vi "Get Recipe Version.vi"(8 "error in (no error)":errorcluster, 11 "Test Recipe in":refnum<class "Test Recipe.lvclass">) -> (0 "error out":errorcluster, 2 "Test Recipe Version":string, 3 "Test Recipe out":refnum<class "Test Recipe.lvclass">)   [LabVIEW 2015, in "Test Recipe.lvlib" / "Test Recipe.lvclass"]
doc: "Searches for a recipe version and retrieves it. Returns \"9.9.9.9\" if no version exists."
uses:
  Test Recipe.lvclass
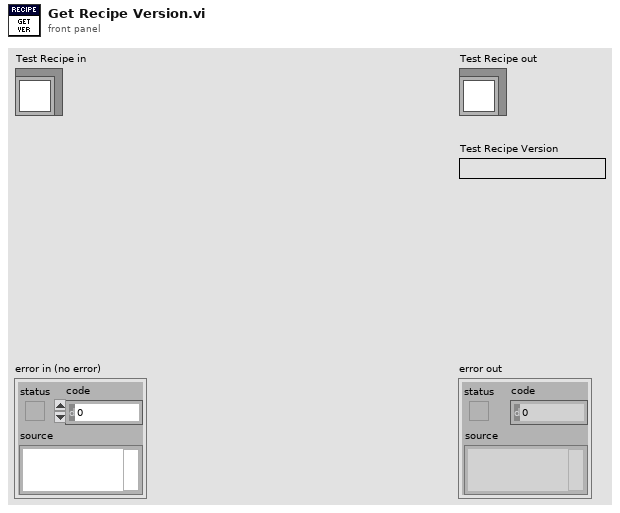
[diagram p1: front panel]
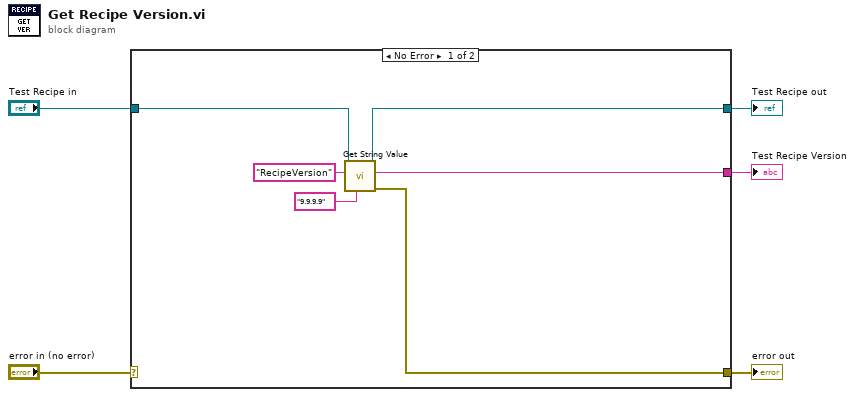
[diagram p0: block diagram]
diagram:
  n1 = case shown="No Error" "error in (no error)" {
    selector: "error in (no error)" -> [_ w13]
    tunnel: [w6 w13] -> w4
    tunnel: [w10 w12] -> w2
    tunnel: "Test Recipe in" -> [w11 w12]
    tunnel: [w7 _] -> w1
    frame No Error {
      n2 = call "Get String Value.vi"("Default Value"="9.9.9.9", "Name"="RecipeVersion", "Test Recipe in"=w11) -> ("error out"=w6:errorcluster, "Value"=w7:string, "Test Recipe out"=w10:refnum<class "Test Recipe.lvclass">)  [unwired: 6 in]
    }
    frame Error {
    }
  }
  "error out" <- w4
  "Test Recipe out" <- w2
  "Test Recipe Version" <- w1
